vi "BroadcastTransmissionPortData.vi"(3 "error in (no error)":errorcluster, 4 "UDP Robot Inputs & Status":T1(array[cluster])=[{"Left Speed (1150 to 1750)"=1500, "Right Speed (1150 to 1750)"=1500, "Robot Heading"=0, "UDP Transmitting Port"=61541, "UDP Receiving Port"=61540, "Robot Symbol"="R"}, {"Left Speed (1150 to 1750)"=1500, "Right Speed (1150 to 1750)"=1500, "Robot Heading"=0, "UDP Transmitting Port"=61543, "UDP Receiving Port"=61542, "Robot Symbol"="G"}, {"Left Speed (1150 to 1750)"=1500, "Right Speed (1150 to 1750)"=1500, "Robot Heading"=0, "UDP Transmitting Port"=61545, "UDP Receiving Port"=61544, "Robot Symbol"="B"}], 5 "connection ID":refnum<k16>) -> (0 "error out":errorcluster, 1 "Data sent":string, 2 "connection ID out":refnum<k16>)   [LabVIEW 2012]
panel:
  out "Example Data Sent (data rec'd)":string="$,R,61541,61540,G,61543,61542,B,61545,61544,S,22,1,349\r"
  # "BROADCAST\nTRANSMISSON\nPORTS"
  # "UDP In"
  # "UDP Out"
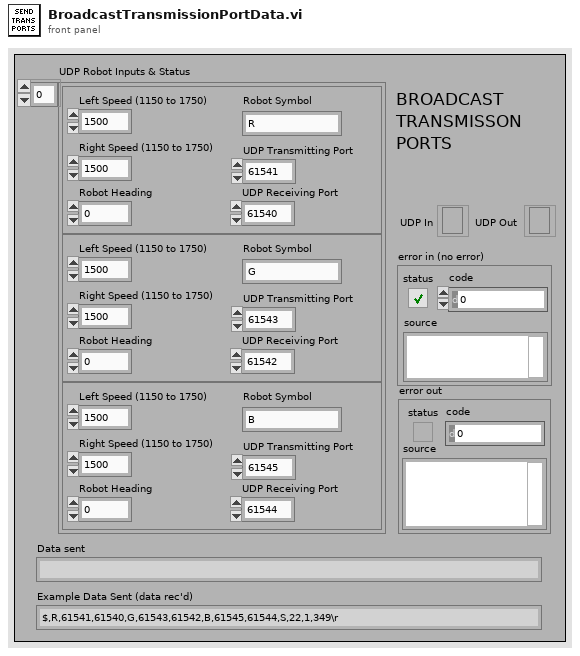
[diagram p1: front panel]
types:
  T1 = cluster{"Left Speed (1150 to 1750)":i32, "Right Speed (1150 to 1750)":i32, "Robot Heading":i32, "UDP Transmitting Port":i32, "UDP Receiving Port":i32, "Robot Symbol":string}[]
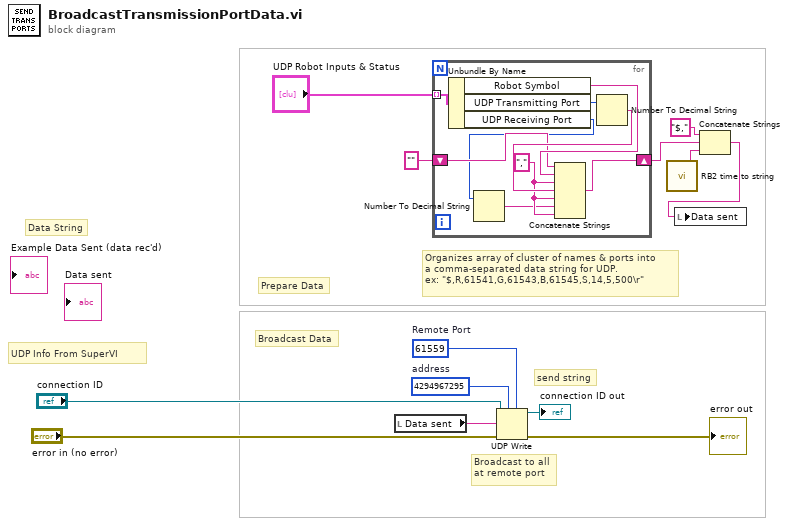
[diagram p0: block diagram]
diagram:
  w9 = u16 61559  # Remote Port
  w8 = u32 4294967295  # address
  # "Data String"
  # "Broadcast Data"
  # "send string"
  # "Broadcast to all\nat remote port"
  # "UDP Info From SuperVI"
  # "Organizes array of cluster of names & ports into\na comma-separated data string for UDP.\nex: \"$,R,61541,G,61543,B,61545,S,14,5,500\\r\""
  # "Prepare Data"
  n1 = local read "Data sent"() -> (w7:string)
  n2 = for {
    tunnel: "UDP Robot Inputs & Status" -> [w22] mode=indexing
    shift-right: [w20] -> w2
    shift-left: "" -> [w17]
    w16 = "," ("string")
    n3 = Unbundle By Name(w22) -> ("Robot Symbol"=w18:string, "UDP Transmitting Port"=w19:i32, "UDP Receiving Port"=w14:i32)
    n4 = Number To Decimal String(number=w14) -> (decimal integer string=w15:string)  [unwired: 1 in]
    n5 = Number To Decimal String(number=w19) -> (decimal integer string=w21:string)  [unwired: 1 in]
    n6 = Concatenate Strings(w17, w18, w16, w21, w16, w15, w16) -> (w20:string)
  }
  n7 = UDP Write(address=w8, port or service name=w9, connection ID="connection ID", data in=w7, 8:"error in (no error)") -> (error out=→"error out":errorcluster, 3:→"connection ID out":refnum<k16>)  [unwired: 1 out]
  n8 = call "RB2 time to string.vi"() -> ("time string"=w10:string)  [unwired: 1 in]
  n9 = Concatenate Strings("$," ("string"), w2, w10) -> (w12:string)
  n10 = local write "Data sent"(w12) -> ()
